vi "Get TSInstall by Version (all architectures).vi"(8 "error in":errorcluster, 10 "Version":string, 11 "ITSDiscovery in":refnum<class "ITSDiscovery.lvclass">) -> (0 "error out":errorcluster, 3 "TSInstall Out":T1)   [LabVIEW 2025]
doc: "This VI retrieves TestStand installations of any architecture."
uses:
  ITSDiscovery/ITSDiscovery.lvclass
  Type Definitions/TSInstall--cluster.ctl
  Type Definitions/Architecture--enum.ctl
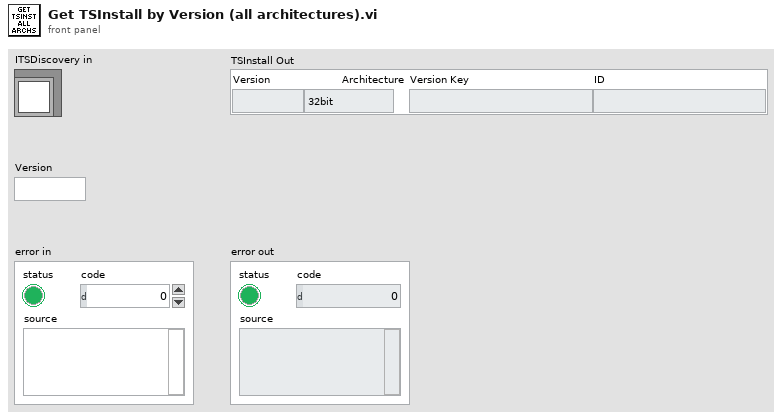
[diagram p1: front panel]
types:
  T1 = typedef "TSInstall--cluster.ctl" = cluster{"Version":string, "Architecture":T2, "Version Key":string, "ID":string}
  T2 = typedef "Architecture--enum.ctl" = enum16{"32bit", "64bit"}
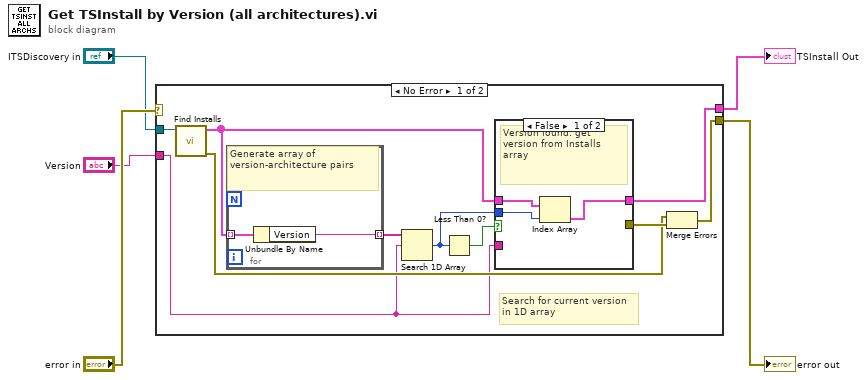
[diagram p0: block diagram]
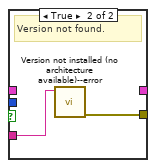
[diagram p2: hidden frame]
diagram:
  n1 = case shown="No Error" "error in" {
    selector: "error in" -> [_ w23]
    tunnel: "ITSDiscovery in" -> [w12 _]
    tunnel: [w13 w23] -> w4
    tunnel: [w8 _] -> w2
    tunnel: "Version" -> [w6 _]
    frame No Error {
      # "Search for current version\nin 1D array"
      n2 = call-dynamic "Find Installs.vi"("ITSDiscovery in"=w12) -> ("error out"=w14:errorcluster, "TSInstalls Out"=w10:T1[])  [unwired: 9 in]
      n3 = for {
        tunnel: w10 -> [w22] mode=indexing
        tunnel: [w21] -> w7 mode=indexing
        # "Generate array of version-architecture pairs"
        n4 = Unbundle By Name(w22) -> ("Version"=w21:string)
      }
      n5 = Search 1D Array(1D array=w7, element=w6) -> (index of element=w9:i32)  [unwired: 1 in]
      n6 = Less Than 0?(x=w9) -> (x < 0?=w11:bool)
      n7 = case shown="False" w11 {
        tunnel: w6 -> [_ w19]
        tunnel: w10 -> [w18 _]
        tunnel: w9 -> [w17 _]
        tunnel: [w16 _] -> w8
        tunnel: [_ w20] -> w15
        frame False {
          # "Version found: get version from Installs array"
          n8 = Index Array(array=w18, index=w17) -> (element=w16:T1)
        }
        frame True {
          # "Version not found."
          n9 = call "Version not installed (no architecture available)--error.vi"("Version"=w19) -> ("error out"=w20:errorcluster)  [unwired: 10 in]
        }
      }
      n10 = Merge Errors(w14, w15) -> (w13:errorcluster)
    }
    frame Error {
      # "Pass error without further action"
    }
  }
  "error out" <- w4
  "TSInstall Out" <- w2
